vi "RFID Get ID  - 2.vi"(11 "ComPort":refnum<visa-resource-name>="COM10") -> (0 "error out":errorcluster, 3 "received":string)   [LabVIEW 2018]
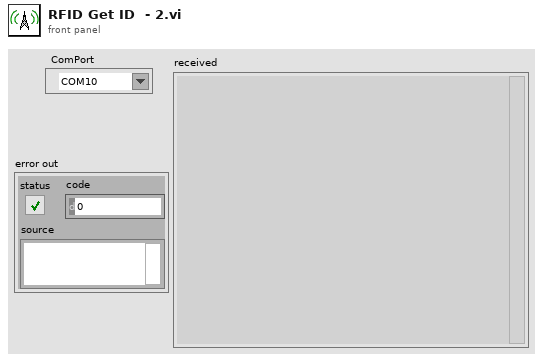
[diagram p1: front panel]
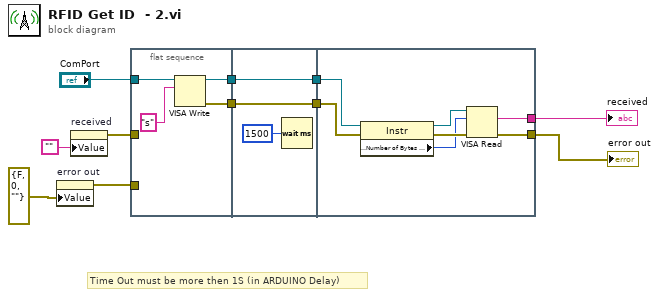
[diagram p0: block diagram]
diagram:
  # "Time Out must be more then 1S (in ARDUINO Delay)"
  n1 = property on="error out" class="Clust (strict)"("Value"=errorcluster {"status"=FALSE, "code"=0, "source"=""} ("error out")) -> (error out=w3:errorcluster)  [unwired: 2 in, 1 out]
  n2 = property on="received" class="Str"("Value"="") -> (error out=w6:errorcluster)  [unwired: 2 in, 1 out]
  n3 = flat-sequence {
    tunnel: "ComPort" -> [w15]
    tunnel: [w13] -> w10
    tunnel: [w12] -> w9
    tunnel: w6 -> [_]
    tunnel: w3 -> [_]
    tunnel: w10 -> [w17]
    tunnel: w9 -> [w16]
    tunnel: [w17] -> w8
    tunnel: [w16] -> w7
    tunnel: w8 -> [w22]
    tunnel: w7 -> [w21]
    tunnel: [w20] -> w2
    tunnel: [w19] -> w1
    frame #0 {
      n4 = VISA Write(VISA resource name=w15, write buffer="s") -> (VISA resource name out=w13:refnum<visa-resource-name>, error out=w12:errorcluster)  [unwired: 1 in, 1 out]
    }
    frame #1 {
      n5 = Wait (ms)(milliseconds to wait=u32 1500) -> ()  [unwired: 1 out]
    }
    frame #2 {
      n6 = property class="Instr"(reference=w22, error in=w21) -> (reference out=w24:refnum<visa-resource-name>, error out=w25:errorcluster, "Serial Settings:Number of Bytes at Serial Port"=w23:u32)
      n7 = VISA Read(VISA resource name=w24, byte count=w23, error in (no error)=w25) -> (read buffer=w19:string, error out=w20:errorcluster)  [unwired: 2 out]
    }
  }
  "received" <- w1
  "error out" <- w2
